vi "Get Target Type.vi"(11 "TimerDRV in":refnum<class "TimerDRV.lvclass">) -> (2 "Target Type":T1, 3 "TimerDRV out":refnum<class "TimerDRV.lvclass">)   [LabVIEW 2019, in "TimingDRV Engine.lvlib" / "TimerDRV.lvclass"]
uses:
  TimerDRV.lvclass
  TypeDefs/Target Type.ctl
  TimerDRV.lvclass/TimerDRV.ctl
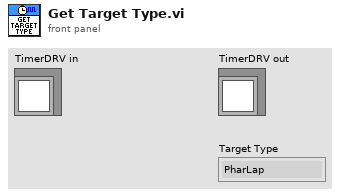
[diagram p1: front panel]
types:
  T1 = typedef "TimingDRV Engine.lvlib/TimerDRV.lvclass/Target Type.ctl" = enum16{"PharLap", "VxWorks", "Windows", "Linux_32_ARM", "Linux_x64"}
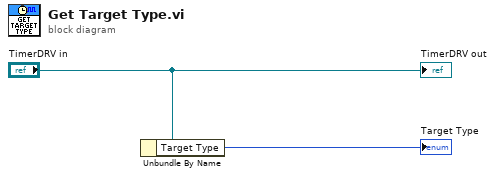
[diagram p0: block diagram]
diagram:
  n1 = Unbundle By Name("TimerDRV in") -> ("Target Type"=→"Target Type":T1)
  "TimerDRV out" <- "TimerDRV in"
